vi "JOSY Binarray Datasocket cmd external.vi"(0 "DataSocketCluster In":T1={"Server Machine"="siskin", "Client Machine"="becard", "Data"="P2", "TimeStamp"=0.0, "Count"=0, "Target Process"="General Server"} {"TimeStamp" format="%.2f"}, 1 "TimeOut Time (s)":dbl=5.0 format="%.2f", 2 "TimeStamp":dbl, 5 "Command":string, 7 "String val":string, 9 "Value":dbl, 11 "error in (no error)":errorcluster, 12 "Command has variable":bool, 13 "Count in":i32, 14 "String":bool) -> (4 "DataSocketCluster Out":T1 {"TimeStamp" format="%.2f"}, 6 "Reply data":string, 10 "Count out":i32, 15 "error out":errorcluster)   [LabVIEW 2020]
uses:
  DataSocketCluster external.ctl
  vi Mode external.ctl
panel:
  # "Notes:\nServer machine: this is always the computer being controlled\nClient machine: this is always the computer doing the controlling - this machine for this example program\nTarget process: this has to match what is coded into the program on the server machine"
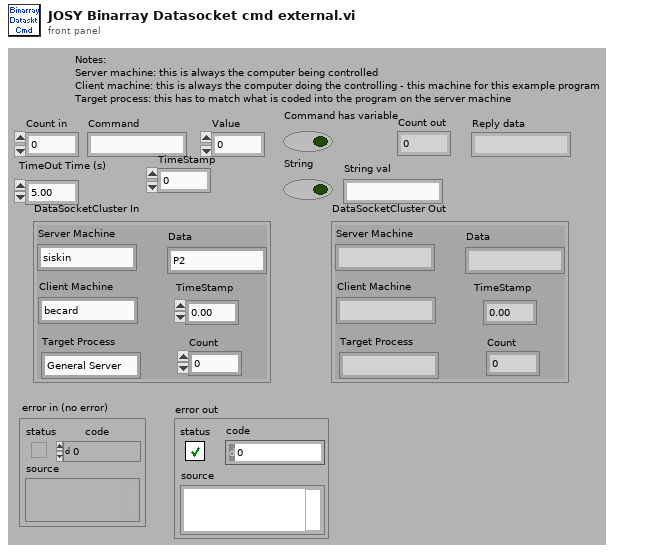
[diagram p1: front panel]
types:
  T1 = typedef "DataSocketCluster external.ctl" = cluster{"Server Machine":string, "Client Machine":string, "Data":string, "TimeStamp":dbl, "Count":i32, "Target Process":string}
  T2 = typedef "vi Mode external.ctl" = enum16{"Client", "Server"}
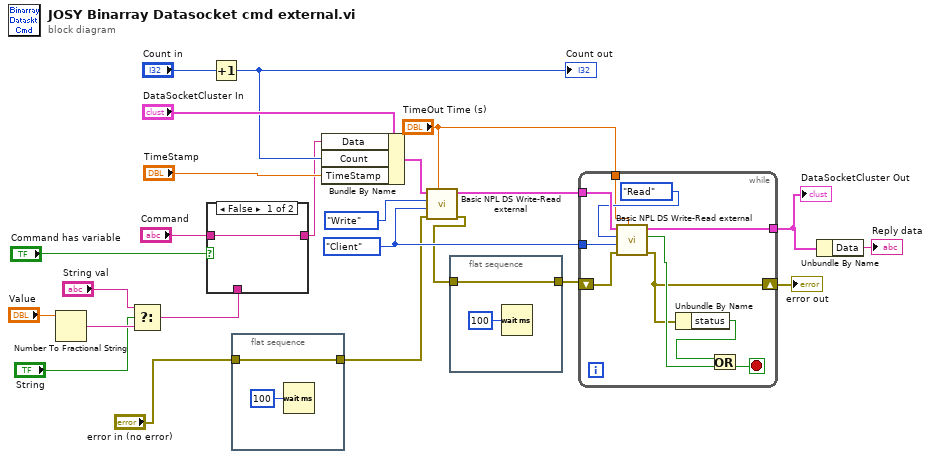
[diagram p0: block diagram]
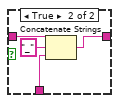
[diagram p2: hidden frame]
diagram:
  w18 = vi_Mode_external."Client" ("Server Mode")
  n1 = Number To Fractional String(number="Value") -> (F-format string=w8:string)  [unwired: 3 out]
  n2 = Select(t="String val", s="String", f=w8) -> (s? t:f=w7:string)
  n3 = case shown="False" "Command has variable" {
    tunnel: "Command" -> [w25 w28]
    tunnel: [w25 w29] -> w11
    tunnel: w7 -> [_ w26]
    frame False {
    }
    frame True {
      n4 = Concatenate Strings(w28, "_", w26) -> (w29:string)
    }
  }
  n5 = Increment(x="Count in") -> (x+1=w21:i32)
  "Count out" <- w21
  n6 = flat-sequence {
    tunnel: "error in (no error)" -> [w31]
    tunnel: [w31] -> w1
    frame #0 {
      n7 = Wait (ms)(milliseconds to wait=u32 100) -> ()  [unwired: 1 out]
    }
  }
  n8 = Bundle By Name(cluster="DataSocketCluster In", "Data"=w11, "Count"=w21, "TimeStamp"="TimeStamp") -> (w16:T1)
  n9 = call "Basic NPL DS Write-Read external.vi"("TimeOut Time (s)"="TimeOut Time (s)", "error in (no error)"=w1, "Server Mode"=w18, "Operation Mode"=enum16{"Read", "Write", "Write/Read"}."Write", "DataSocketCluster In"=w16) -> ("error out"=w4:errorcluster, "DataSocketCluster Out"=w19:T1)  [unwired: 3 out]
  n10 = flat-sequence {
    tunnel: w4 -> [w33]
    tunnel: [w33] -> w3
    frame #0 {
      n11 = Wait (ms)(milliseconds to wait=u32 100) -> ()  [unwired: 1 out]
    }
  }
  n12 = while {
    shift-right: [w36] -> w24
    shift-left: w3 -> [w43]
    tunnel: w19 -> [w42]
    tunnel: w18 -> [w40]
    tunnel: "TimeOut Time (s)" -> [w38]
    tunnel: [w37] -> w10
    stop <- w35 stop-if-true
    n13 = call "Basic NPL DS Write-Read external.vi"("TimeOut Time (s)"=w38, "error in (no error)"=w43, "Server Mode"=w40, "Operation Mode"=enum16{"Read", "Write", "Write/Read"}."Read", "DataSocketCluster In"=w42) -> ("error out"=w36:errorcluster, "New Data"=w41:bool, "DataSocketCluster Out"=w37:T1)  [unwired: 2 out]
    n14 = Unbundle By Name(w36) -> ("status"=w34:bool)
    n15 = Or(x=w34, y=w41) -> (x .or. y?=w35:bool)
  }
  "error out" <- w24
  "DataSocketCluster Out" <- w10
  n16 = Unbundle By Name(w10) -> ("Data"=→"Reply data":string)
